vi "Initialise Default Cube.vi"(8 "error in (no error)":errorcluster, 11 "Resource Directory":path) -> (0 "error out":errorcluster, 3 "Cube":T1 {"Triangles"."Vertex 3"."UV"."v" min=0 max=1 step=0.1; "Triangles"."Vertex 3"."UV"."u" min=0 max=1 step=0.1; "Triangles"."Vertex 2"."UV"."v" min=0 max=1 step=0.1; "Triangles"."Vertex 2"."UV"."u" min=0 max=1 step=0.1; "Triangles"."Vertex 1"."UV"."v" min=0 max=1 step=0.1; "Triangles"."Vertex 1"."UV"."u" min=0 max=1 step=0.1})   [LabVIEW 2020, in "Application.lvlib" / "Scene.lvclass"]
uses:
  Scene.lvclass
  Libraries/3D/Object.ctl
  Libraries/3D/Triangle.ctl
  Libraries/3D/Vertex.ctl
  Libraries/3D/Vector 3D.ctl
  Libraries/Raster/UV.ctl
  Libraries/3D/Material.ctl
  Libraries/Raster/Texture.ctl
  Libraries/Raster/Rectangle Dimensions.ctl
  Libraries/3D/Transform.ctl
  Libraries/3D/3D.lvlib
  Libraries/Raster/Raster.lvlib
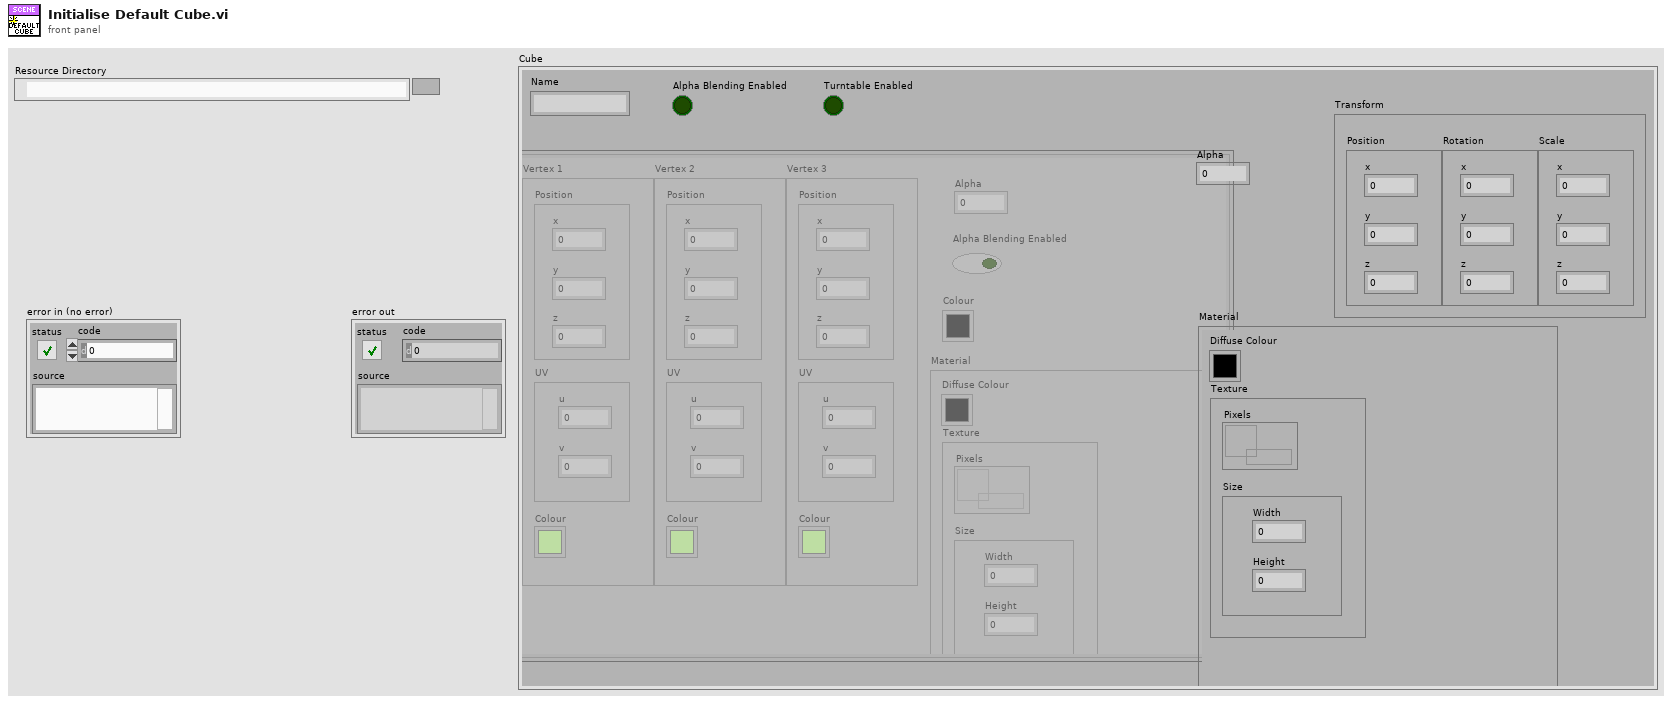
[diagram p1: front panel]
types:
  T1 = typedef "3D.lvlib/Object.ctl" = cluster{"Triangles":T2[], "Transform":T9, "Name":string, "Alpha Blending Enabled":bool, "Alpha":dbl, "Turntable Enabled":bool, "Material":T6}
  T2 = typedef "3D.lvlib/Triangle.ctl" = cluster{"Vertex 1":T3, "Vertex 2":T3, "Vertex 3":T3, "Alpha":dbl, "Alpha Blending Enabled":bool, "Colour":u32, "Material":T6}
  T3 = typedef "3D.lvlib/Vertex.ctl" = cluster{"Position":T4, "UV":T5, "Colour":u32}
  T4 = typedef "3D.lvlib/Vector 3D.ctl" = cluster{"x":sgl, "y":sgl, "z":sgl}
  T5 = typedef "Raster.lvlib/UV.ctl" = cluster{"u":sgl, "v":sgl}
  T6 = typedef "3D.lvlib/Material.ctl" = cluster{"Diffuse Colour":u32, "Texture":T7}
  T7 = typedef "Raster.lvlib/Texture.ctl" = cluster{"Pixels":refnum<data-value>, "Size":T8}
  T8 = typedef "Raster.lvlib/Rectangle Dimensions.ctl" = cluster{"Width":u32, "Height":u32}
  T9 = typedef "3D.lvlib/Transform.ctl" = cluster{"Position":T4, "Rotation":T4, "Scale":T4}
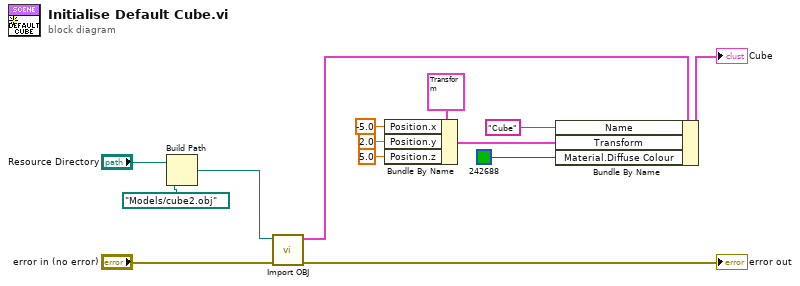
[diagram p0: block diagram]
diagram:
  n1 = Build Path(base path="Resource Directory", name or relative path=path "Models/cube2.obj") -> (appended path=w3:path)
  n2 = call "Import OBJ.vi"("error in (no error)"="error in (no error)", "Object"=w3) -> ("error out"=→"error out":errorcluster, "Object"=w5:T1)  [unwired: 8 in]
  n3 = Bundle By Name(cluster=T9 {"Position"={"x"=2.0, "y"=1.0, "z"=-5.0}, "Rotation"={"x"=0.0, "y"=0.0, "z"=0.0}, "Scale"={"x"=0.0, "y"=0.0, "z"=0.0}} ("Transform"), "Position.x"=sgl -5.0, "Position.y"=sgl 2.0, "Position.z"=sgl 5.0) -> (w8:T9)
  n4 = Bundle By Name(cluster=w5, "Name"="Cube", "Transform"=w8, "Material.Diffuse Colour"=u32 242688 ("Diffuse Colour")) -> (→"Cube":T1)
